vi "resize.vi"(6 "Height":u32=400, 7 "Width":u32=500, 9 "Pane 4":refnum<vi>, 10 "reference out 2":refnum<vi>, 11 "Pane in":refnum<vi>) -> (3 "reference out":refnum<vi>)   [LabVIEW 2020]
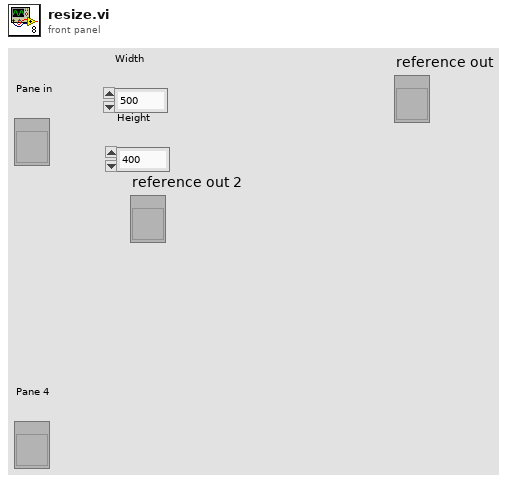
[diagram p1: front panel]
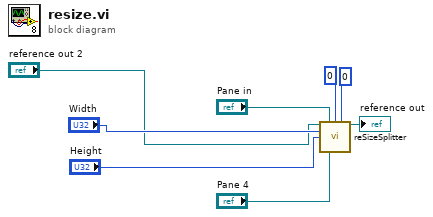
[diagram p0: block diagram]
diagram:
  n1 = call "reSizeSplitter.vi"("this vi"="reference out 2", "pane"="Pane in", "left"=i16 0, "top"=i16 0, "Width"="Width", "Height"="Height", "pane2"="Pane 4") -> ("reference out"=→"reference out":refnum<vi>)  [unwired: 8 in]
